vi "Agilent SNA Set Trigger Mode.vi"(6 "Channel":i8=1 min=1 max=99 step=1, 7 "Agilent SNA & SWP":T1, 8 "error in (no error)":errorcluster, 10 "Trigger Mode":T2, 11 "VISA Resource Names":T3) -> (0 "error out":errorcluster, 3 "dup VISA Resource Names":T3)   [LabVIEW 2011]
doc: "This VI for the HP8753B Network Analyzers reads the stimulus values. Except when performing log sweeps and freq list sweeps, this VI uses the start and stop values and the number of points to calcuate the stimulus values."
uses:
  TypeDefs/Agilent SNA VISA.ctl
  TypeDefs/Agilent SNA Trigger Mode.ctl
  TypeDefs/Agilent SNA Instrument Info.ctl
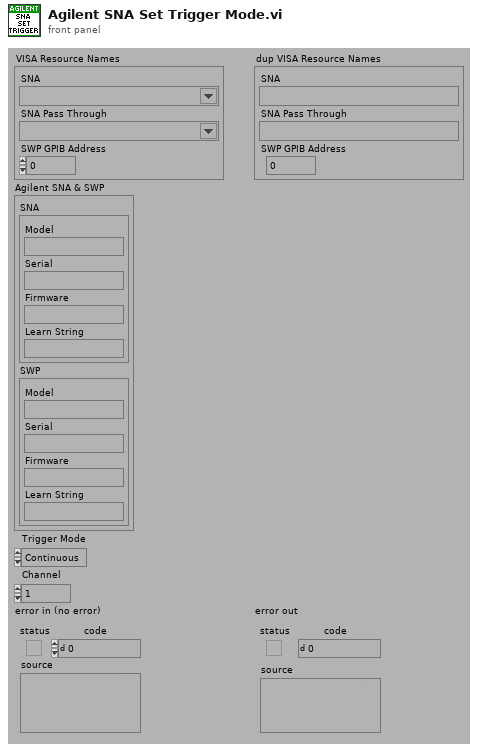
[diagram p1: front panel]
types:
  T1 = typedef "Agilent SNA Instrument Info.ctl" = cluster{"SNA":cluster{"Model":string, "Serial":string, "Firmware":string, "Learn String":string}, "SWP":cluster{"Model":string, "Serial":string, "Firmware":string, "Learn String":string}}
  T2 = typedef "Agilent SNA Trigger Mode.ctl" = enum16{"Continuous", "Hold", "Single"}
  T3 = typedef "Agilent SNA VISA.ctl" = cluster{"SNA":refnum<visa-resource-name>, "SNA Pass Through":refnum<visa-resource-name>, "SWP GPIB Address":i32}
  T4 = typedef "Agilent SNA Model.ctl" = enum16{"Not Supported", "8757X"}
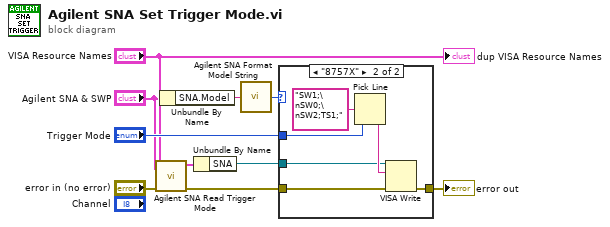
[diagram p0: block diagram]
diagram:
  n1 = call "Agilent SNA Read Trigger Mode.vi"("Agilent SNA & SWP"="Agilent SNA & SWP", "error in (no error)"="error in (no error)", "VISA Resource Names"="VISA Resource Names") -> ("error out"=w7:errorcluster, "dup VISA Resource Names"=w4:T3)  [unwired: 1 in, 6 out]
  n2 = Unbundle By Name("Agilent SNA & SWP") -> ("SNA.Model"=w6:string)
  n3 = Unbundle By Name(w4) -> ("SNA"=w3:refnum<visa-resource-name>)
  n4 = call "Agilent SNA Format Model String.vi"("Model String"=w6) -> ("Model"=w5:T4)
  n5 = case shown="\"8757X\"" w5 {
    tunnel: [w11 w12] -> w10
    tunnel: "Trigger Mode" -> [_ w13]
    tunnel: w7 -> [w11 w15]
    tunnel: w3 -> [_ w14]
    frame "Not Supported" {
    }
    frame "8757X" {
      n6 = Pick Line(multi-line string="SW1;\nSW0;\nSW2;TS1;", line index=w13) -> (output string=w17:string)  [unwired: 1 out]
      n7 = VISA Write(VISA resource name=w14, write buffer=w17, error in (no error)=w15) -> (error out=w12:errorcluster)  [unwired: 2 out]
    }
  }
  "error out" <- w10
  "dup VISA Resource Names" <- "VISA Resource Names"
